vi "StepperController.vi"() -> ()   [LabVIEW 2020]
panel:
  in  "D":u16(ring)=13 items=["DIO0", "DIO1", "DIO2", "DIO3", "DIO4", "DIO5", "DIO6", "DIO7", "EIO0", "EIO1", "EIO2", "EIO3", "EIO4", "EIO5", "EIO6", "EIO7", "CIO0", "CIO1", "CIO2", "CIO3", "MIO0", "MIO1", "MIO2"]
  in  "C":u16(ring)=12 items=["DIO0", "DIO1", "DIO2", "DIO3", "DIO4", "DIO5", "DIO6", "DIO7", "EIO0", "EIO1", "EIO2", "EIO3", "EIO4", "EIO5", "EIO6", "EIO7", "CIO0", "CIO1", "CIO2", "CIO3", "MIO0", "MIO1", "MIO2"]
  in  "B":u16(ring)=9 items=["DIO0", "DIO1", "DIO2", "DIO3", "DIO4", "DIO5", "DIO6", "DIO7", "EIO0", "EIO1", "EIO2", "EIO3", "EIO4", "EIO5", "EIO6", "EIO7", "CIO0", "CIO1", "CIO2", "CIO3", "MIO0", "MIO1", "MOI2"]
  in  "A":u16(ring)=8 items=["DIO0", "DIO1", "DIO2", "DIO3", "DIO4", "DIO5", "DIO6", "DIO7", "EIO0", "EIO1", "EIO2", "EIO3", "EIO4", "EIO5", "EIO6", "EIO7", "CIO0", "CIO1", "CIO2", "CIO3", "MIO0", "MIO1", "MIO2"]
  in  "Zero?":bool
  in  "Program":enum16{"FULL STEP", "HALF STEP"}(ring)
  in  "GUAGE STOP":bool
  in  "Mode Select":bool=TRUE
  in  "Gauge Control Mode":dbl(knob) scale=0.0..200.0
  out "Position":dbl=100.0
  in  "ARRAY STOP":bool
  in  "Wait Between Steps (ms)":dbl=1500.0
  in  "Steps/Rotation":dbl=200.0
  in  "Array Control Mode":dbl[](array[numeric])=[0.0, 50.0, 100.0, 150.0, 200.0, 150.0, 100.0, 50.0, 0.0, 400.0, 0.0]
  out "error out":errorcluster
  out "Error String":string="No Error"
  in  "error in (no error)":errorcluster
  out "ConnectionType Out":i32=1
  out "DeviceType Out":i32=4
  in  "Identifier":string="LJM_idANY"
  in  "Connection Type":string="LJM_ctANY"
  in  "Device Type":string="LJM_dtANY"
  # "Before use, select the corect stepper channels, program, steps/rotation of the stepper, and wait\nbetween steps for array mode. If using array mode, also fill the control array. Then, select either\ngauge or array mode and run the VI. While  in gauge mode, select reset/zero to set a new home."
  # "Channel Select"
  # "Gauge"
  # "Array"
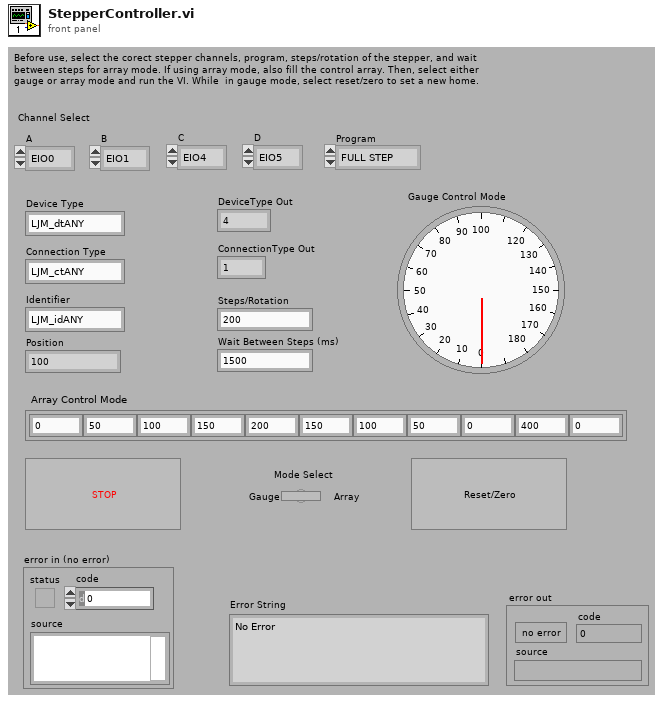
[diagram p1: front panel]
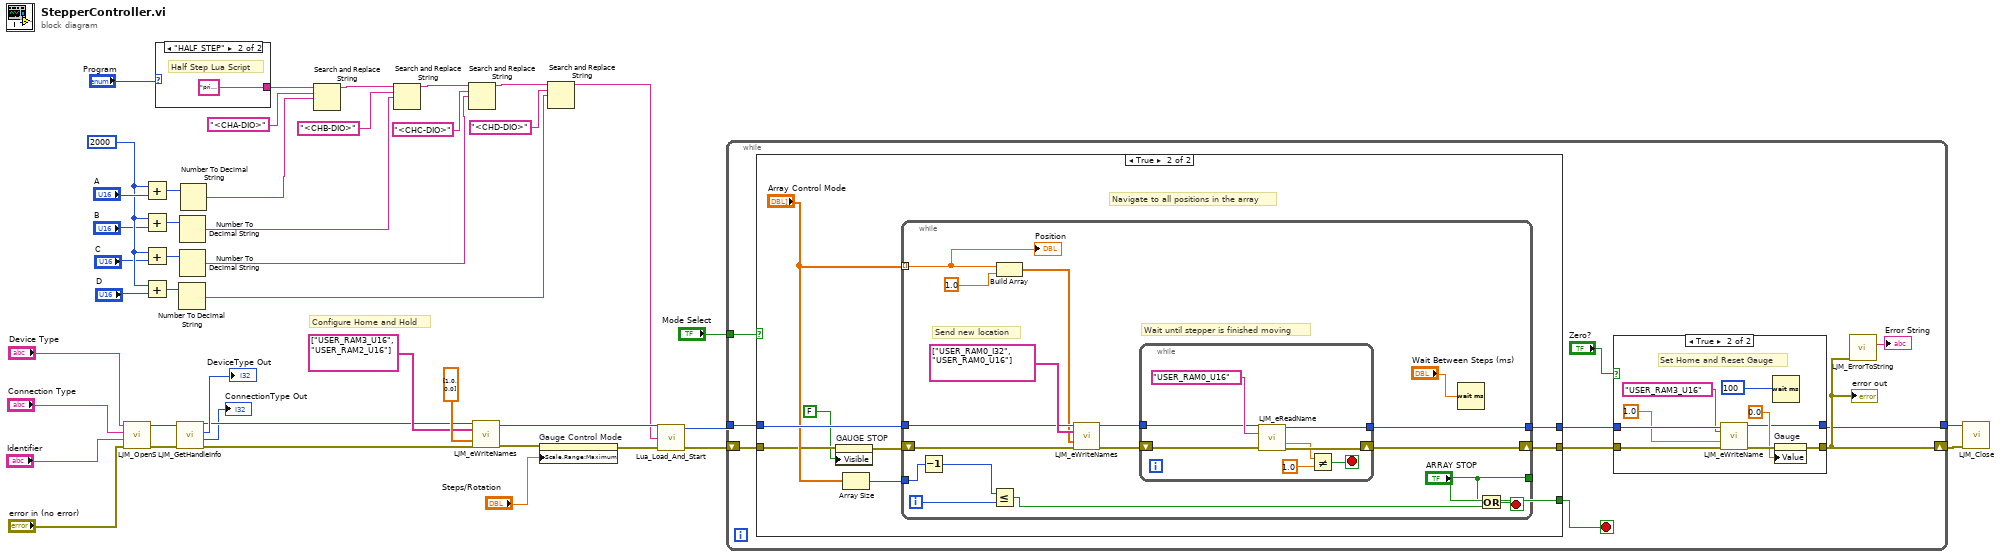
[diagram p0: block diagram]
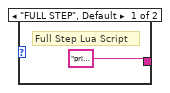
[diagram p2: hidden frame]
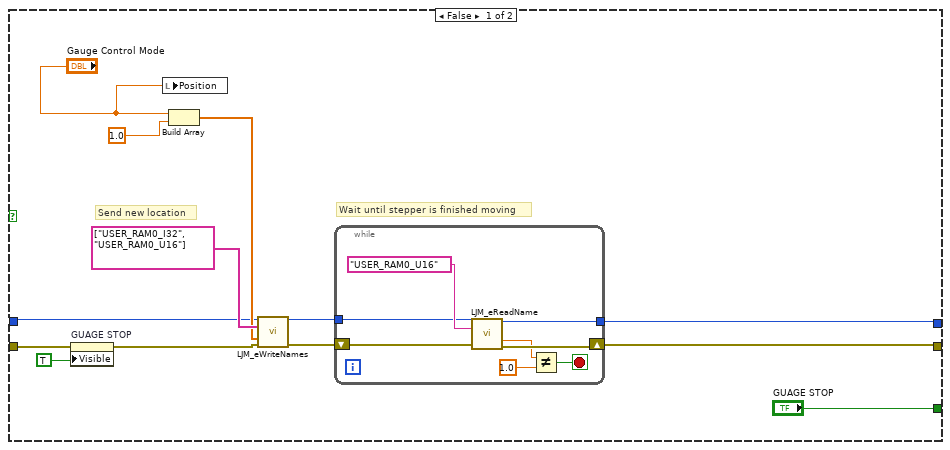
[diagram p4: hidden frame]
diagram:
  w12 = 2000
  # "Configure Home and Hold"
  n1 = call "LJM_OpenS.vi"("error in"="error in (no error)", "Identifier"="Identifier", "ConnectionType"="Connection Type", "DeviceType"="Device Type") -> ("error out"=w43:errorcluster, "Handle"=w42:i32)  [unwired: 6 in]
  n2 = Add(x=w12, y="A") -> (x+y=w11:i32)
  n3 = Add(x=w12, y="B") -> (x+y=w10:i32)
  n4 = Add(x=w12, y="C") -> (x+y=w9:i32)
  n5 = Add(x=w12, y="D") -> (x+y=w8:i32)
  n6 = case shown="\"HALF STEP\"" "Program" {
    tunnel: ["print(\"Use the following registers:\")\nprint(\"46080: Target Position (steps)\")\nprint(\"46082: Current Position (steps)\")\n\nprint(\"46180: enable, 1:enable, 0: disable\")print(\"46181: eStop, 1: eStop, 0: run\")\nprint(\"46182: hold, 1: hold position of motor, 0: release motor (after movement)\")\nprint(\"46183: setHome, (setHome)\")\n\nlocal mbR = MB.R\nlocal mbW = MB.W\n\n-- Configurable Variables\n\nlocal enable = false -- 46180, \"USER_RAM0_U16\", type: 0;\nlocal targ = 0 -- 46080, \"USER_RAM1_I32\", type: 2\nlocal pos = 0 -- 46082, \"USER_RAM0_I32\", type: 2 enable/disable control.\nlocal eStop = 0 -- 46181, \"USER_RAMx_U16\", type: 0; Value read before setting I/O line states to immediately disengage motor.\nlocal hold = 1 -- 46184, \"USER_RAMx_U16\", type: 0;Enable hold mode by default at end of movement sequence.\nlocal setHome = 0 -- 46184, \"USER_RAM0_U16\", type: 0; Set new \"zero\" or \"home\"\n\n\n-- Define FIO Channels\nlocal chA = <CHA-DIO>\nlocal chB = <CHB-DIO>\nlocal chC = <CHC-DIO>\nlocal chD = <CHD-DIO>\nmbW(chA, 0, 0) --EIO0 =  DIO8\nmbW(chB, 0, 0) --EIO1 =  DIO9\nmbW(chC, 0, 0) --EIO4 = DIO12\nmbW(chD, 0, 0) --EIO5 = DIO13\n\n--Define the Full Step Sequence\nlocal a = {1,0,0,0}\nlocal b = {0,0,1,0}\nlocal c = {0,1,0,0}\nlocal d = {0,0,0,1}\nlocal numSteps =table.getn(a)\n\nlocal i = 0\nlocal m0, m1, m2, m3 = 0\n\n-- Set initial USER_RAM values.\nmbW(46080, 2, targ)\nmbW(46082, 2, pos)\n\nmbW(46180, 0, enable)\nmbW(46181, 0, eStop)\nmbW(46182, 0, hold)\nmbW(46183, 0, setHome) -- Initialize variable used for the Re-Zero \"target\"/Motor control.\n\nLJ.IntervalConfig(0, 4) -- For stepper motor control\nLJ.IntervalConfig(1, 1000) -- For printing current state\n\nwhile true do\n  if LJ.CheckInterval(1) then\n    print(\"Current State\", enable, target, pos, eStop)\n  end\n\n  if LJ.CheckInterval(0) then\n\n    enable = (mbR(46180, 0) == 1) -- Determine if we should start moving.\n    targ = mbR(46080, 2) -- Read desired \"target\"\n\n    if enable then -- if allowed to move\n      if pos == targ then--if we have reached the new position\n\n        --write enable to 0 to signal finished\n        enable = false\n        mbW(46180, 0, 0)\n\n        print(\"reached new pos\")\n\n        -- Determine if motor should be \"held in place\"\n        hold = mbR(46182, 0)\n        if hold == 0 then\n          --set all low to allow free movement\n          m0 = 0\n          m1 = 0\n          m2 = 0\n          m3 = 0\n        end\n        --else if hold then keep the same position activated\n        \n      elseif pos < targ then -- if behind, go foreward\n        pos = pos+1--increment position by 1\n        i = pos%numSteps+1--lua is 1-indexed, so add a 1\n        \n        m0 = a[i]--write the new positions\n        m1 = b[i]\n        m2 = c[i]\n        m3 = d[i]\n        \n      elseif pos > targ then-- if ahead, move back\n        pos = pos-1\n        i = pos%numSteps+1\n        \n        m0 = a[i]\n        m1 = b[i]\n        m2 = c[i]\n        m3 = d[i]\n      end\n    else -- if not enable\n      hold = mbR(46182, 0)\n      setHome = mbR(46183, 0)\n\n      if setHome == 1 then-- if home register is set to make a new home\n        print(\"New home created\")\n        mbW(46183, 0, 0)\n        pos = 0;--make a new home\n      end\n\n      if hold == 0 then\n        m0 = 0\n        m1 = 0\n        m2 = 0\n        m3 = 0\n      end\n    end\n\n    -- Update variable with current position\n    mbW(46082, 2, pos)\n\n    eStop = mbR(46181, 0)\n    if eStop == 1 then\n      m0 = 0; m1 = 0; m2 = 0; m3 = 0\n    end\n\n    mbW(chA, 0, m0) --EIO0 =  DIO8\n    mbW(chB, 0, m1) --EIO1 =  DIO9\n    mbW(chC, 0, m2) --EIO2 = DIO10\n    mbW(chD, 0, m3) --EIO3 = DIO11\n  end\nend" "print(\"Use the following registers:\")\nprint(\"46080: Target Position (steps)\")\nprint(\"46082: Current Position (steps)\")\n\nprint(\"46180: enable, 1:enable, 0: disable\")\nprint(\"46181: eStop, 1: eStop, 0: run\")\nprint(\"46182: hold, 1: hold position of motor, 0: release motor (after movement)\")\nprint(\"46183: setHome, (setHome)\")\n\nlocal mbR = MB.R\nlocal mbW = MB.W\n\n-- Configurable Variables\nlocal targ = 0 -- 46080, \"USER_RAM1_I32\", type: 2\nlocal pos = 0 -- 46082, \"USER_RAM0_I32\", type: 2\n\nlocal enable = false -- 46180, \"USER_RAM0_U16\", type: 0; enable/disable control.\nlocal eStop = 0 -- 46181, \"USER_RAMx_U16\", type: 0; Value read before setting I/O line states to immediately disengage motor.\nlocal hold = 1 -- 46184, \"USER_RAMx_U16\", type: 0;Enable hold mode by default at end of movement sequence.\nlocal setHome = 0 -- 46184, \"USER_RAM0_U16\", type: 0; Set new \"zero\" or \"home\"\n\n\n-- Define FIO Channels\nlocal chA = <CHA-DIO>\nlocal chB = <CHB-DIO>\nlocal chC = <CHC-DIO>\nlocal chD = <CHD-DIO>\nmbW(chA, 0, 0) --EIO0 =  DIO8\nmbW(chB, 0, 0) --EIO1 =  DIO9\nmbW(chC, 0, 0) --EIO4 = DIO12\nmbW(chD, 0, 0) --EIO5 = DIO13\n\n--Define the Half Step Sequence\nlocal a = {1,1,0,0,0,0,0,1}\nlocal b = {0,0,0,1,1,1,0,0}\nlocal c = {0,1,1,1,0,0,0,0}\nlocal d = {0,0,0,0,0,1,1,1}\nlocal numSteps =table.getn(a)\n\nlocal i = 0\nlocal m0, m1, m2, m3 = 0\n\n-- Set initial USER_RAM values.\nmbW(46080, 2, targ)\nmbW(46082, 2, pos)\n\nmbW(46180, 0, enable)\nmbW(46181, 0, eStop)\nmbW(46182, 0, hold)\nmbW(46183, 0, setHome) -- Initialize variable used for the Re-Zero \"target\"/Motor control.\n\nLJ.IntervalConfig(0, 4) -- For stepper motor control\nLJ.IntervalConfig(1, 1000) -- For printing current state\n\nwhile true do\n  if LJ.CheckInterval(1) then\n    print(\"Current State\", enable, target, pos, eStop)\n  end\n\n  if LJ.CheckInterval(0) then\n\n    enable = (mbR(46180, 0) == 1) -- Determine if we should start moving.\n    targ = mbR(46080, 2) -- Read desired \"target\"\n\n    if enable then -- if allowed to move\n      if pos == targ then--if we have reached the new position\n\n        --write enable to 0 to signal finished\n        enable = false\n        mbW(46180, 0, 0)\n\n        print(\"reached new pos\")\n\n        -- Determine if motor should be \"held in place\"\n        hold = mbR(46182, 0)\n        if hold == 0 then\n          --set all low to allow free movement\n          m0 = 0\n          m1 = 0\n          m2 = 0\n          m3 = 0\n        end\n        --else if hold then keep the same position activated\n        \n      elseif pos < targ then -- if behind, go foreward\n        pos = pos+1--increment position by 1\n        i = pos%numSteps+1--lua is 1-indexed, so add a 1\n        \n        m0 = a[i]--write the new positions\n        m1 = b[i]\n        m2 = c[i]\n        m3 = d[i]\n        \n      elseif pos > targ then-- if ahead, move back\n        pos = pos-1\n        \n        i = pos%numSteps+1\n        m0 = a[i]\n        m1 = b[i]\n        m2 = c[i]\n        m3 = d[i]\n      end\n    else -- if not enable\n      hold = mbR(46182, 0)\n      setHome = mbR(46183, 0)\n\n      if setHome == 1 then-- if home register is set to make a new home\n        print(\"New home created\")\n        mbW(46183, 0, 0)\n        pos = 0;--make a new home\n      end\n\n      if hold == 0 then\n        m0 = 0\n        m1 = 0\n        m2 = 0\n        m3 = 0\n      end\n    end\n\n    -- Update variable with current position\n    mbW(46082, 2, pos)\n\n    eStop = mbR(46181, 0)\n    if eStop == 1 then\n      m0 = 0; m1 = 0; m2 = 0; m3 = 0\n    end\n\n    mbW(chA, 0, m0) --EIO0 =  DIO8\n    mbW(chB, 0, m1) --EIO1 =  DIO9\n    mbW(chC, 0, m2) --EIO2 = DIO10\n    mbW(chD, 0, m3) --EIO3 = DIO11\n  end\nend"] -> w22
    frame "FULL STEP", Default {
      # "Full Step Lua Script"
    }
    frame "HALF STEP" {
      # "Half Step Lua Script"
    }
  }
  n7 = call "LJM_GetHandleInfo.vi"("error in"=w43, "Handle In"=w42) -> ("error out"=w37:errorcluster, "ConnectionType"=→"ConnectionType Out":i32, "DeviceType"=→"DeviceType Out":i32, "Handle Out"=w29:i32)  [unwired: 2 in, 4 out]
  n8 = Number To Decimal String(number=w8) -> (decimal integer string=w1:string)  [unwired: 1 in]
  n9 = Number To Decimal String(number=w10) -> (decimal integer string=w3:string)  [unwired: 1 in]
  n10 = Number To Decimal String(number=w9) -> (decimal integer string=w2:string)  [unwired: 1 in]
  n11 = Number To Decimal String(number=w11) -> (decimal integer string=w4:string)  [unwired: 1 in]
  n12 = Search and Replace String(input string=w22, search string="<CHA-DIO>", replace string=w4) -> (result string=w21:string)  [unwired: 5 in, 3 out]
  n13 = Search and Replace String(input string=w21, search string="<CHB-DIO>", replace string=w3) -> (result string=w20:string)  [unwired: 5 in, 3 out]
  n14 = Search and Replace String(input string=w20, search string="<CHC-DIO>", replace string=w2) -> (result string=w19:string)  [unwired: 5 in, 3 out]
  n15 = call "LJM_eWriteNames.vi"("Handle In"=w29, "aNames"=string[] ["USER_RAM3_U16", "USER_RAM2_U16"], "aValuesIn"=dbl[] [1.0, 0.0], "error in"=w37) -> ("Handle Out"=w24:i32, "error out"=w30:errorcluster)  [unwired: 9 in, 1 out]
  n16 = property on="Gauge Control Mode" class="Knob (strict)"(error in=w30, "Scale.Range:Maximum"="Steps/Rotation") -> (error out=w25:errorcluster)  [unwired: 1 in, 1 out]
  n17 = Search and Replace String(input string=w19, search string="<CHD-DIO>", replace string=w1) -> (result string=w14:string)  [unwired: 5 in, 3 out]
  n18 = call "Lua_Load_And_Start.vi"("error in (no error)"=w25, "Lua Script"=w14, "Handle In"=w24) -> ("error out"=w26:errorcluster, "Handle Out"=w27:i32)  [unwired: 1 out]
  n19 = while {
    shift-right: [w49] -> w35
    shift-left: w26 -> [w56]
    tunnel: "Mode Select" -> [w54]
    tunnel: w27 -> [w55]
    tunnel: [w48] -> w32
    stop <- w53 stop-if-true
    n20 = case shown="True" w54 {
      tunnel: w56 -> [w70 w91]
      tunnel: w55 -> [w74 w97]
      tunnel: [w73 w96] -> w51
      tunnel: [w72 w95] -> w50
      tunnel: ["GUAGE STOP" w92] -> w53
      frame False {
        # "Send new location"
        # "Wait until stepper is finished moving"
        n21 = property on="GUAGE STOP" class="Bool"(error in=w70, "Visible"=TRUE) -> (error out=w69:errorcluster)  [unwired: 1 in, 1 out]
        n22 = local write "Position"("Gauge Control Mode") -> ()
        n23 = Build Array("Gauge Control Mode", 1.0) -> (w78:dbl[])
        n24 = call "LJM_eWriteNames.vi"("Handle In"=w74, "aNames"=string[] ["USER_RAM0_I32", "USER_RAM0_U16"], "aValuesIn"=w78, "error in"=w69) -> ("Handle Out"=w76:i32, "error out"=w77:errorcluster)  [unwired: 9 in, 1 out]
        n25 = while {
          shift-right: [w87] -> w72
          shift-left: w77 -> [w88]
          tunnel: w76 -> [w85]
          tunnel: [w82] -> w73
          stop <- w81 stop-if-true
          n26 = call "LJM_eReadName.vi"("Handle In"=w85, "Name"="USER_RAM0_U16", "error in"=w88) -> ("Handle Out"=w82:i32, "Value"=w84:dbl, "error out"=w87:errorcluster)  [unwired: 10 in]
          n27 = Not Equal?(x=w84, y=1.0) -> (x != y?=w81:bool)
        }
      }
      frame True {
        # "Navigate to all positions in the array"
        n28 = property on="GAUGE STOP" class="Bool"(error in=w91, "Visible"=FALSE) -> (error out=w90:errorcluster)  [unwired: 1 in, 1 out]
        n29 = Array Size(array="Array Control Mode") -> (size(s)=w93:i32)
        n30 = while {
          tunnel: w97 -> [w112]
          tunnel: [w106] -> w96
          shift-right: [w108] -> w95
          shift-left: w90 -> [w113]
          tunnel: "Array Control Mode" -> [w101] mode=indexing
          tunnel: w93 -> [w104]
          tunnel: ["ARRAY STOP"] -> w92
          i -> [w99]
          stop <- w103 stop-if-true
          # "Send new location"
          # "Wait until stepper is finished moving"
          n31 = Decrement(x=w104) -> (x-1=w100:i32)
          n32 = Less Or Equal?(x=w100, y=w99) -> (x <= y?=w98:bool)
          n33 = Build Array(w101, 1.0) -> (w110:dbl[])
          n34 = call "LJM_eWriteNames.vi"("Handle In"=w112, "aNames"=string[] ["USER_RAM0_I32", "USER_RAM0_U16"], "aValuesIn"=w110, "error in"=w113) -> ("Handle Out"=w107:i32, "error out"=w109:errorcluster)  [unwired: 9 in, 1 out]
          n35 = while {
            shift-right: [w121] -> w108
            shift-left: w109 -> [w122]
            tunnel: w107 -> [w119]
            tunnel: [w116] -> w106
            stop <- w115 stop-if-true
            n36 = call "LJM_eReadName.vi"("Handle In"=w119, "Name"="USER_RAM0_U16", "error in"=w122) -> ("Handle Out"=w116:i32, "Value"=w118:dbl, "error out"=w121:errorcluster)  [unwired: 10 in]
            n37 = Not Equal?(x=w118, y=1.0) -> (x != y?=w115:bool)
          }
          n38 = Wait (ms)(milliseconds to wait="Wait Between Steps (ms)") -> ()  [unwired: 1 out]
          n39 = Or(x="ARRAY STOP", y=w98) -> (x .or. y?=w103:bool)
          "Position" <- w101
        }
      }
    }
    n40 = case shown="True" "Zero?" {
      tunnel: w51 -> [w58 w67]
      tunnel: w50 -> [w57 w66]
      tunnel: [w57 w62] -> w49
      tunnel: [w58 w60] -> w48
      frame False {
      }
      frame True {
        # "Set Home and Reset Gauge"
        n41 = call "LJM_eWriteName.vi"("Handle In"=w67, "Name"="USER_RAM3_U16", "Value"=1.0, "error in"=w66) -> ("Handle Out"=w60:i32, "error out"=w63:errorcluster)  [unwired: 10 in]
        n42 = Wait (ms)(milliseconds to wait=100) -> ()  [unwired: 1 out]
        n43 = property on="Gauge" class="Knob (strict)"(error in=w63, "Value"=0.0) -> (error out=w62:errorcluster)  [unwired: 1 in, 1 out]
      }
    }
    "error out" <- w49
    n44 = call "LJM_ErrorToString.vi"("error in"=w49) -> ("String"=→"Error String":string)  [unwired: 10 in]
  }
  n45 = call "LJM_Close.vi"("error in"=w35, "Handle"=w32) -> ()  [unwired: 9 in, 1 out]
